vi "LJM process new open.vi"(8 "error in":errorcluster, 9 "Open New Device?":bool=TRUE, 10 "Open Configs":T1, 11 "Handle":i32) -> (0 "error out":errorcluster, 1 "ConnType":i32, 2 "DevType":i32, 3 "Handle Out":i32, 4 "SerialNumber":i32)   [LabVIEW 2025]
panel:
  out "error out 2":errorcluster
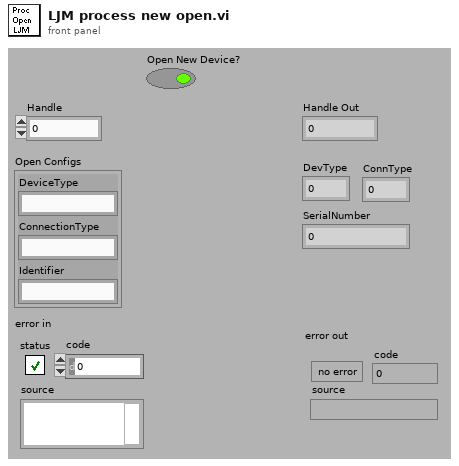
[diagram p1: front panel]
types:
  T1 = cluster{"DeviceType":string, "ConnectionType":string, "Identifier":string}
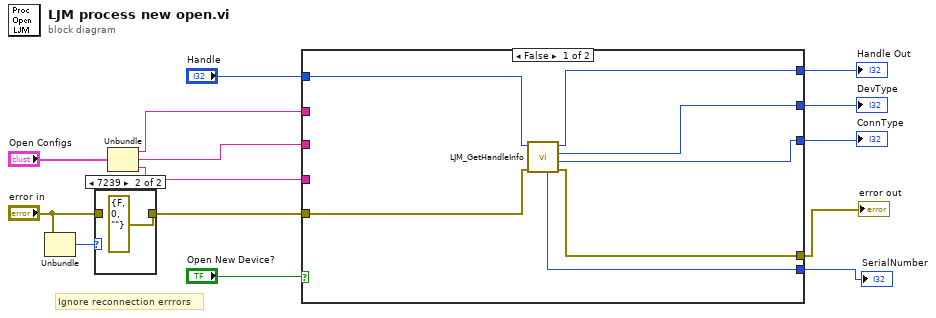
[diagram p0: block diagram]
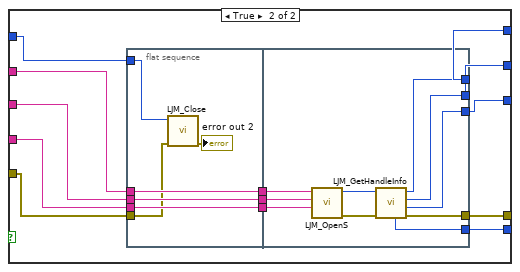
[diagram p3: hidden frame]
diagram:
  # "Ignore reconnection errrors"
  n1 = Unbundle("error in") -> ("code"=w3:i32)  [unwired: 2 out]
  n2 = case shown="7239" w3 {
    tunnel: "error in" -> [w15 _]
    tunnel: [w15 errorcluster {"status"=FALSE, "code"=0, "source"=""} ("error in")] -> w1
    frame 0, Default {
    }
    frame 7239 {
    }
  }
  n3 = Unbundle("Open Configs") -> ("DeviceType"=w6:string, "ConnectionType"=w5:string, "Identifier"=w4:string)
  n4 = case shown="False" "Open New Device?" {
    tunnel: w5 -> [_ w36]
    tunnel: w4 -> [_ w35]
    tunnel: w1 -> [w17 w34]
    tunnel: w6 -> [_ w33]
    tunnel: [w23 w32] -> w14
    tunnel: "Handle" -> [w22 w28]
    tunnel: [w21 w27] -> w11
    tunnel: [w20 w26] -> w10
    tunnel: [w19 w25] -> w9
    tunnel: [w18 w24] -> w8
    frame False {
      n5 = call "LJM_GetHandleInfo.vi"("error in"=w17, "Handle In"=w22) -> ("error out"=w23:errorcluster, "ConnectionType"=w19:i32, "DeviceType"=w20:i32, "Handle Out"=w21:i32, "SerialNumber"=w18:i32)  [unwired: 2 in, 3 out]
    }
    frame True {
      n6 = flat-sequence {
        tunnel: w33 -> [w40]
        tunnel: w34 -> [w38]
        tunnel: w35 -> [w41]
        tunnel: w36 -> [w42]
        tunnel: [w42] -> w31
        tunnel: [w41] -> w30
        tunnel: [w40] -> w29
        tunnel: w28 -> [w39]
        tunnel: [w47] -> w32
        tunnel: w31 -> [w51]
        tunnel: w30 -> [w50]
        tunnel: w29 -> [w49]
        tunnel: [w46] -> w27
        tunnel: [w45] -> w26
        tunnel: [w44] -> w25
        tunnel: [w43] -> w24
        frame #0 {
          n7 = call "LJM_Close.vi"("error in"=w38, "Handle"=w39) -> ("error out"=→"error out 2":errorcluster)  [unwired: 9 in]
        }
        frame #1 {
          n8 = call "LJM_OpenS.vi"("Identifier"=w50, "ConnectionType"=w51, "DeviceType"=w49) -> ("error out"=w48:errorcluster, "Handle"=w52:i32)  [unwired: 7 in]
          n9 = call "LJM_GetHandleInfo.vi"("error in"=w48, "Handle In"=w52) -> ("error out"=w47:errorcluster, "ConnectionType"=w44:i32, "DeviceType"=w45:i32, "Handle Out"=w46:i32, "SerialNumber"=w43:i32)  [unwired: 2 in, 3 out]
        }
      }
    }
  }
  "DevType" <- w10
  "ConnType" <- w9
  "SerialNumber" <- w8
  "Handle Out" <- w11
  "error out" <- w14
